vi "labviewArduino_2.vi"() -> ()   [LabVIEW 2017]
uses:
  <vilib>/MakerHub/LINX/Public/Peripherals/Digital/Digital Write N Chans.vi
  <vilib>/MakerHub/LINX/Private/Local IO/LinxDigitalWrite.vi
  <vilib>/MakerHub/LINX/Public/Utilities/Check Channel.vi
  <vilib>/MakerHub/LINX/Public/Utilities/Open Serial.vi
  <vilib>/MakerHub/LINX/Private/Utilties/Generate Error.vi
  Keithley 24XX/Public/Data/Read (Multiple Points).vi
  <vilib>/Utility/file.llb/Write To Spreadsheet File (DBL).vi
  <vilib>/MakerHub/LINX/LMH-LINX.lvlib
  Keithley 24XX/Keithley 24XX.lvlib
panel:
  in  "Tab Control":enum32{"Settings", "General"}(tab)
  in  "Keithley 2400 Cluster":T1={"Compliance  Level (1)"=1.0, "Number of Points (80)"=80, "Minimum Voltage (-0,1)"=-0.1, "Maximum Voltage (0,7)"=0.7, "Timeout (10000 ms)"=100000, "Keithley 2400 GPIB"="", "Source Mode  (0: Voltage)"=0} {"Source Mode  (0: Voltage)" items=["Voltage", "Current"]; "Timeout (10000 ms)" format="%#.6g"}
  in  "HV-Source Cluster":T2={"Control Mode (T = CV, F = CC)"=TRUE, "CH1 ON/OFF (T = ON)"=FALSE, "CH2 ON/OFF (T = ON)"=FALSE, "CH1 VOLTAGE SET (-2000...0 V)"=0, "CH2 VOLTAGE SET (0...+2000 V)"=0, "CH1 CURRENT SET (0...5 mA)"=5.0, "CH2 CURRENT SET (0...5 mA)"=5.0, "COM Port HV Source"=""} {"CH2 CURRENT SET (0...5 mA)" min=0.0 max=5.0 step=0.1 format="%_4f"; "CH1 CURRENT SET (0...5 mA)" min=0.0 max=5.0 step=0.1 format="%_4f"; "CH2 VOLTAGE SET (0...+2000 V)" min=0 max=2000 step=100; "CH1 VOLTAGE SET (-2000...0 V)" min=-2000 max=0 step=100}
  in  "Switch matrix Cluster":T3={"Switch Matrix Port"="", "High voltage Source polarity"=enum."Not inverted", "Total time High Voltage Source is active (min)"=10.0, " Time between measurements(min)"=5.0, "Amount of modules connected"=enum."1", "path to folder for measuring data"=path "C:/Users/Jorne/Documents/Steering Switch matrix/LabVIEW-Masterproef/data", "Stressed time"=0.0}
  in  "Resume Button":bool
  in  "Stop Button 2":bool
  in  "Start Button":bool
  out "Dark IV curve last measurement":cluster{"Voltage":sgl[], "Current":sgl[]}(graph)
  out "Panel measuring":dbl
  out "Total time(s)":dbl
  out "Stressed time (min)":dbl
  in  "Pauze Button":bool
  in  "HV Source emergency STOP)":bool
  out "Last Rsh (Ohm)":dbl
  out "output Rsh":dbl[][](array[numeric])
  out "Rsh curve over time":cluster{"array":dbl[], "array":dbl[]}(graph)
  # "CURE toevoegen: na de stresstijd een curetijd ingeven\nde naam van de opslagbestanden moet dan ook aangepast?\nbutton voor wel of niet curen"
  # "Pauze knop, als erop wordt gedrukt, stopt het stressen en wanneer er terug op start wordt gedrukt, dan start het programma terug van waar het was gestopt"
  # "interface pimpen, met mooiere indeling en greyed out buttons"
  # "Keithley 2400 Setup"
  # "HV Source Setup"
  # "Switch Matrix Setup"
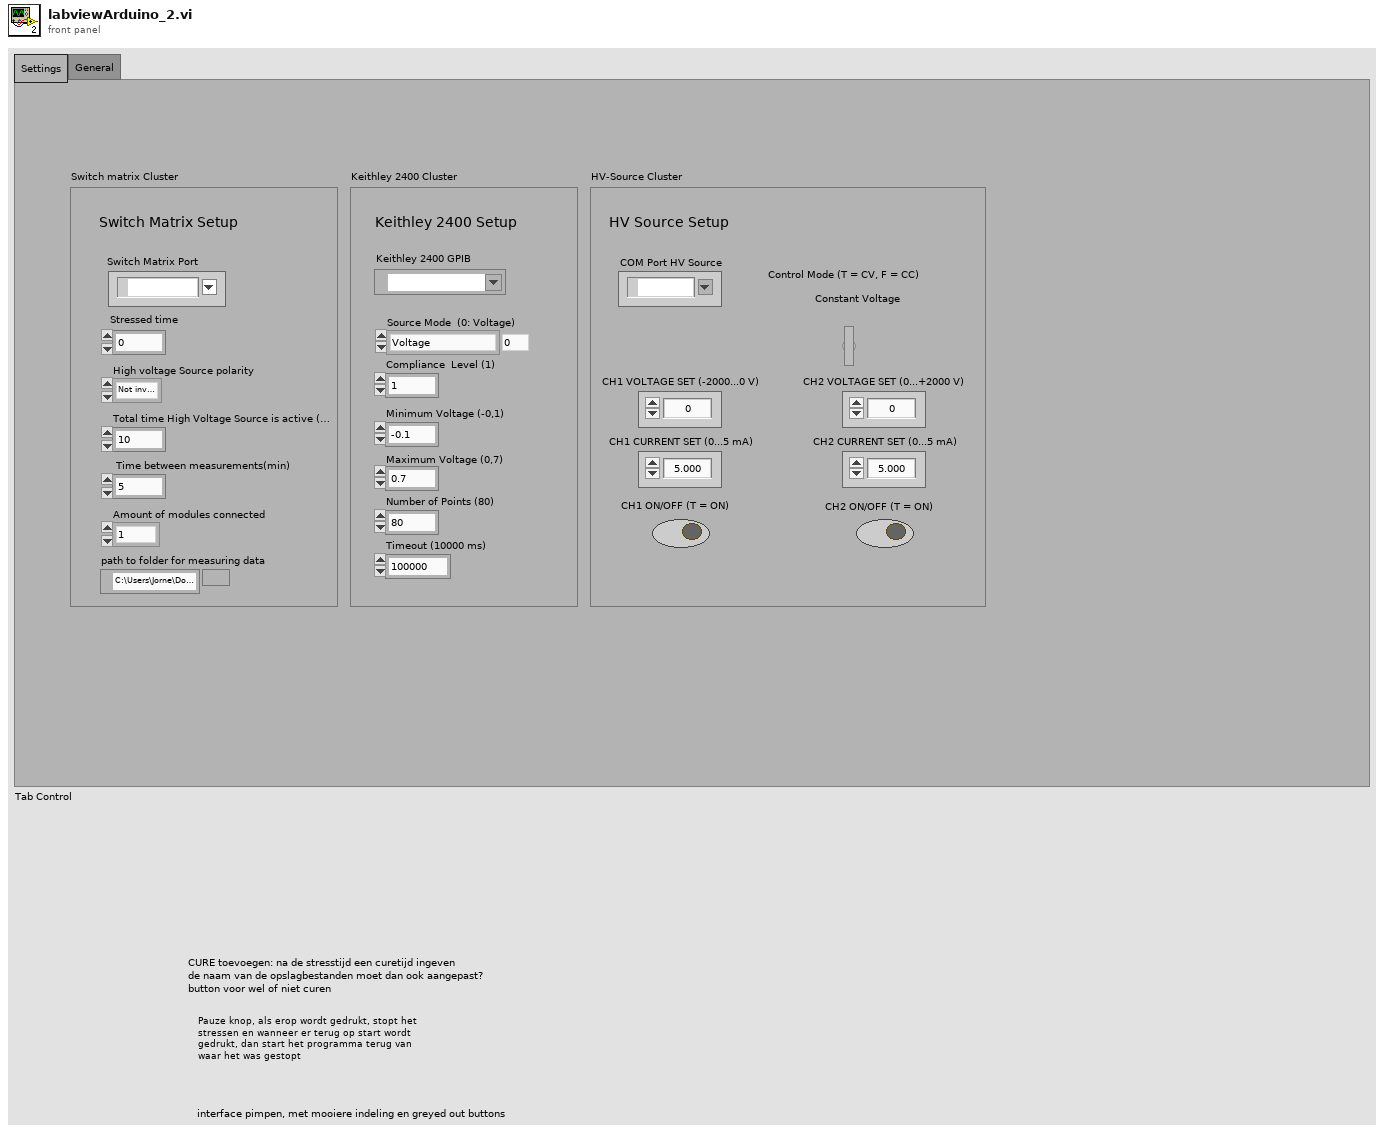
[diagram p1: front panel]
types:
  T1 = cluster{"Compliance  Level (1)":dbl, "Number of Points (80)":u32, "Minimum Voltage (-0,1)":dbl, "Maximum Voltage (0,7)":dbl, "Timeout (10000 ms)":i32, "Keithley 2400 GPIB":refnum<visa-resource-name>, "Source Mode  (0: Voltage)":u16}
  T2 = cluster{"Control Mode (T = CV, F = CC)":bool, "CH1 ON/OFF (T = ON)":bool, "CH2 ON/OFF (T = ON)":bool, "CH1 VOLTAGE SET (-2000...0 V)":i16, "CH2 VOLTAGE SET (0...+2000 V)":i16, "CH1 CURRENT SET (0...5 mA)":dbl, "CH2 CURRENT SET (0...5 mA)":dbl, "COM Port HV Source":refnum<visa-resource-name>}
  T3 = cluster{"Switch Matrix Port":refnum<visa-resource-name>, "High voltage Source polarity":enum16{"Not inverted", "Inverted"}, "Total time High Voltage Source is active (min)":dbl, " Time between measurements(min)":dbl, "Amount of modules connected":enum16{"1", "2", "3", "4", "5", "6"}, "path to folder for measuring data":path, "Stressed time":dbl}
  T4 = enum8{"Enabled", "Disabled", "Disabled and Grayed Out"}
  T5 = enum16{"Rest", "HV Source On", "Measure", "Relay 1", "Relay 2", "Relay 3", "Relay 4", "Relay 5", "Relay 6"}
  T6 = enum16{"Rest", "HV Source On", "Relay 1", "Relay 2", "Relay 3", "Relay 4", "Relay 5", "Relay 6"}
  T7 = typedef "LMH-LINX.lvlib/LINX Ref.ctl" = cluster{"IO":T8, "Interface":T9, "LINX Device Config":T10}
  T8 = typedef "LMH-LINX.lvlib/Platform.ctl" = enum16{"Remote", "Local"}
  T9 = typedef "LMH-LINX.lvlib/Interface.ctl" = enum16{"Serial", "TCP"}
  T10 = typedef "LMH-LINX.lvlib/Device.lvlib/LINX Device Config.ctl" = cluster{"Interface":T9, "COM Port":refnum<visa-resource-name>, "TCP Configuration":T11, "Device Family":u8, "Device ID":u8, "Device Name":string, "TCP Ref":refnum<k5>, "Channels":T12}
  T11 = typedef "LMH-LINX.lvlib/Device.lvlib/TCP Config.ctl" = cluster{"IP Address":string, "Port":u16}
  T12 = typedef "LMH-LINX.lvlib/Channels.ctl" = cluster{"DI":u8[], "DO":u8[], "AI":u8[], "AO":u8[], "PWM":u8[], "QE":u8[], "UART":u8[], "I2C 2":u8[], "SPI":u8[], "CAN":u8[], "Servo":u8[], "AI Ref (V)":dbl, "AI Resolution (Bits)":u8, "AO Ref (V)":dbl, "AO Resolution (Bits)":u8}
  T13 = cluster{"Baud Rate":u32, "Parity":u16, "Data Bits":u16, "Stop Bits":u16, "Flow Control":u16}
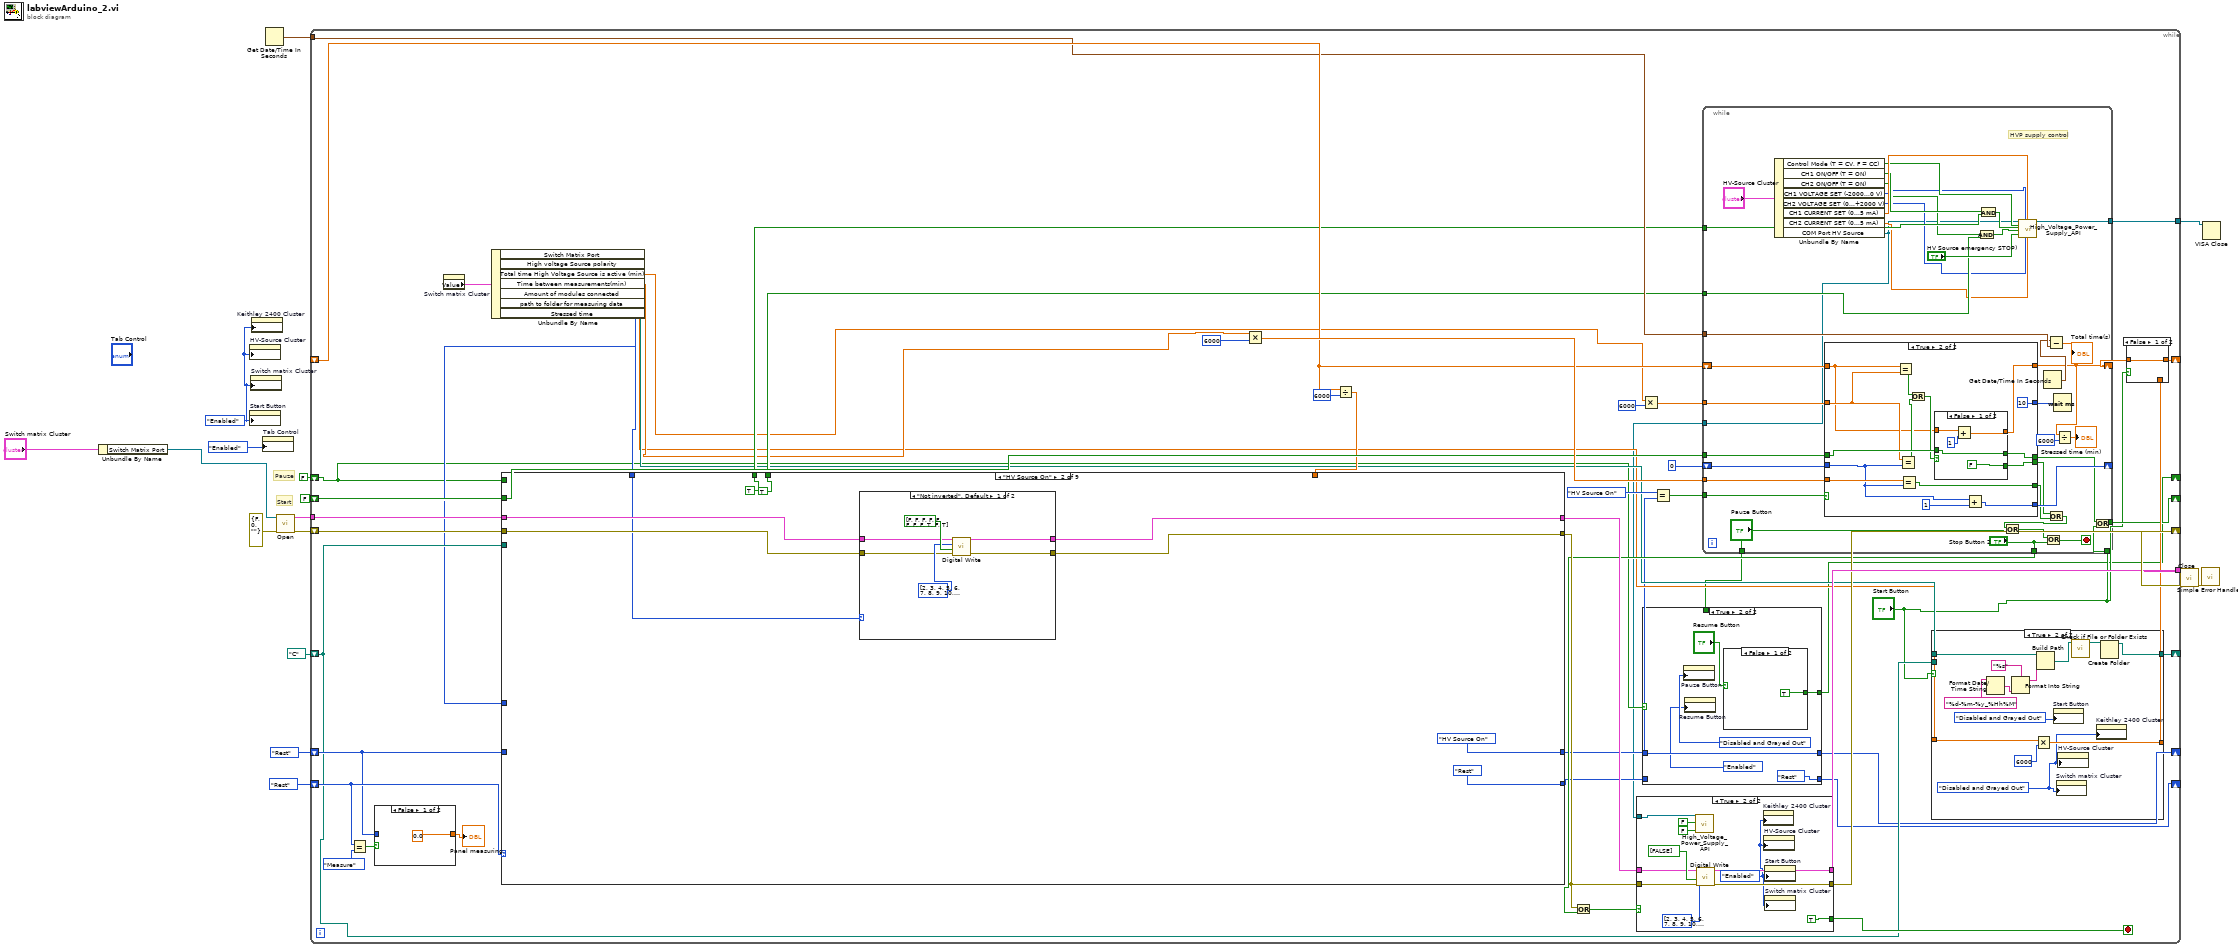
[diagram p0: block diagram]
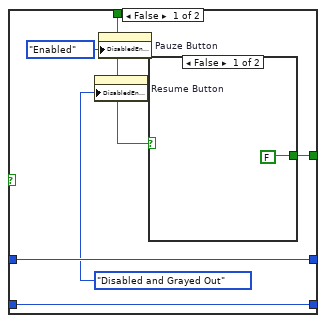
[diagram p2: hidden frame]
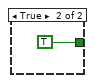
[diagram p3: hidden frame]
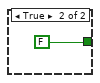
[diagram p4: hidden frame]
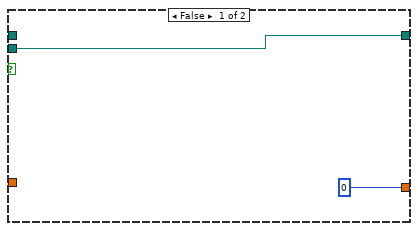
[diagram p6: hidden frame]
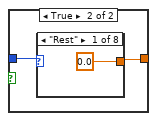
[diagram p7: hidden frame]
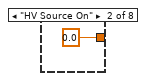
[diagram p8: hidden frame]
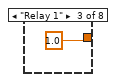
[diagram p9: hidden frame]
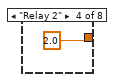
[diagram p10: hidden frame]
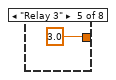
[diagram p11: hidden frame]
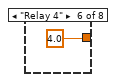
[diagram p12: hidden frame]
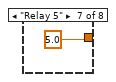
[diagram p13: hidden frame]
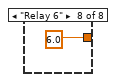
[diagram p14: hidden frame]
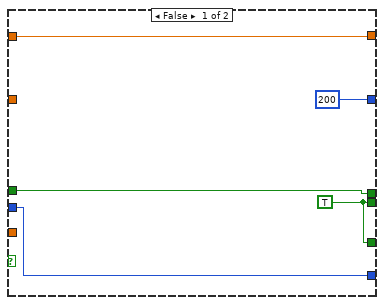
[diagram p15: hidden frame]
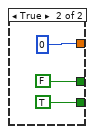
[diagram p16: hidden frame]
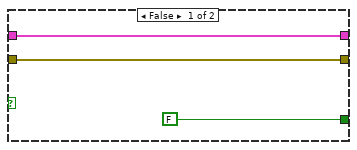
[diagram p17: hidden frame]
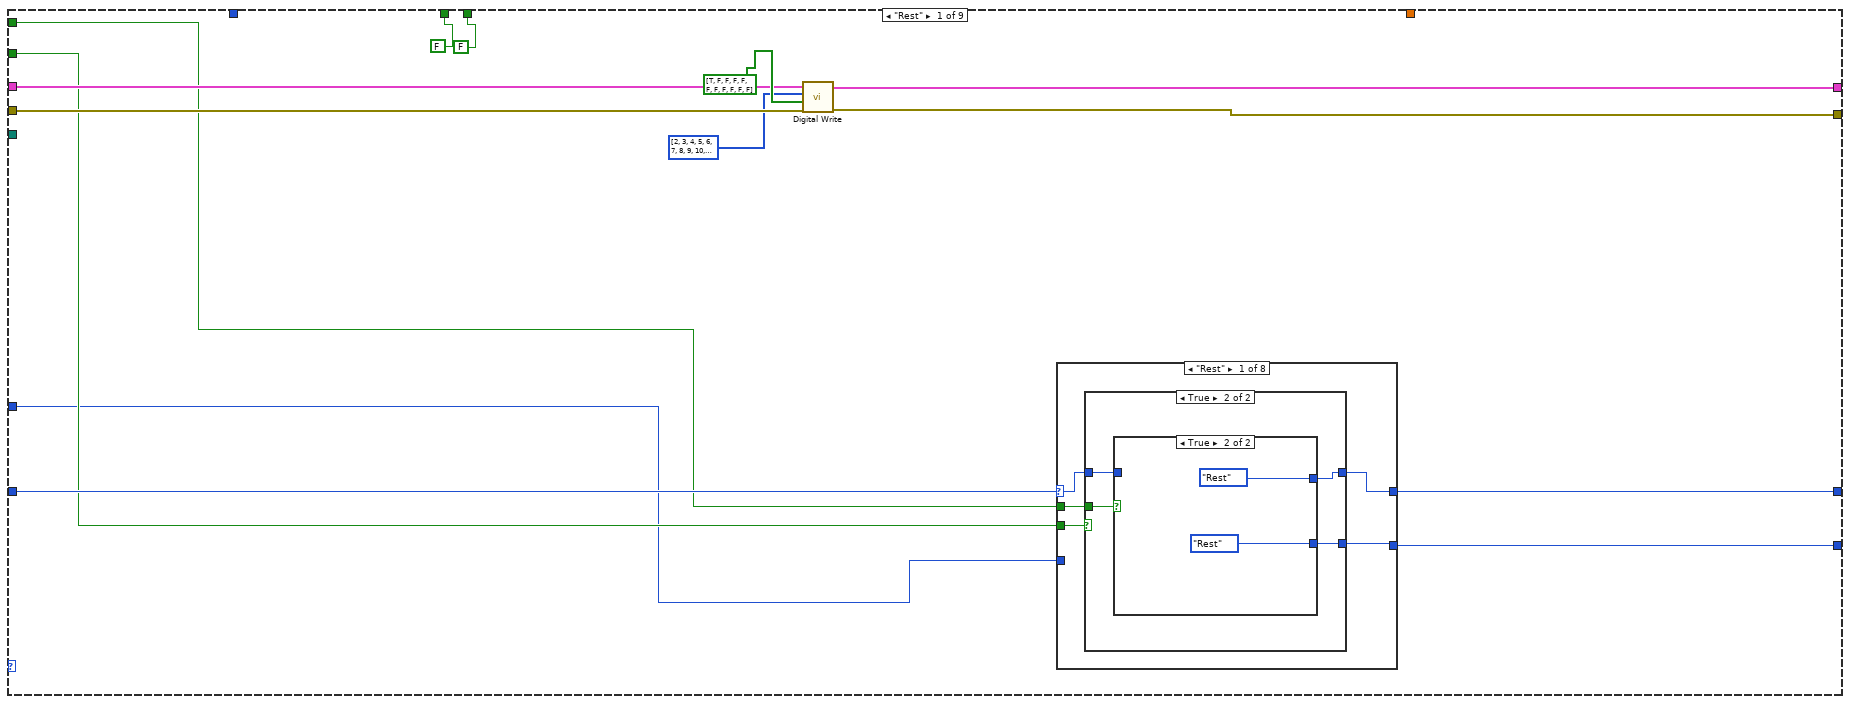
[diagram p18: hidden frame]
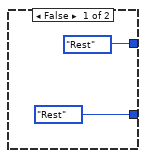
[diagram p19: hidden frame]
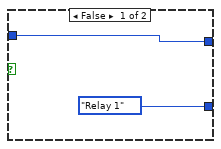
[diagram p20: hidden frame]
diagram:
  w1 = T4."Enabled" ("Disabled")
  # "Start"
  # "Pauze"
  n1 = Unbundle By Name("Switch matrix Cluster") -> ("Switch Matrix Port"=w4:refnum<visa-resource-name>)
  n2 = property on="HV-Source Cluster" class="Clust (strict)"("DisabledEnum"=w1) -> ()  [unwired: 2 in, 2 out]
  n3 = property on="Start Button" class="Bool"("DisabledEnum"=w1) -> ()  [unwired: 2 in, 2 out]
  n4 = property on="Switch matrix Cluster" class="Clust (strict)"("DisabledEnum"=w1) -> ()  [unwired: 2 in, 2 out]
  n5 = property on="Keithley 2400 Cluster" class="Clust (strict)"("DisabledEnum"=w1) -> ()  [unwired: 2 in, 2 out]
  n6 = property on="Tab Control" class="TabCtl (strict)"("DisabledEnum"=T4."Enabled" ("Disabled")) -> ()  [unwired: 2 in, 2 out]
  n7 = Get Date/Time In Seconds() -> (seconds since 1Jan1904=w8:timestamp)
  n8 = call-poly <vilib>:"Open.vi"("Error In"=errorcluster {"status"=FALSE, "code"=0, "source"=""}, "Serial Port"=w4) -> ("Error Out"=w16:errorcluster, "LINX Resource"=w17:T7)  [unwired: 7 in, 1 out]
  n9 = while {
    tunnel: w17 -> [w68]
    tunnel: [w63] -> w15
    shift-right: [w62] -> w14
    shift-left: w16 -> [w67]
    shift-right: [w24] -> _
    shift-left: T5."Rest" ("Enum 2") -> [w49]
    shift-right: [w27] -> _
    shift-left: T6."Rest" ("Enum 2") -> [w46]
    shift-right: [w32] -> _
    shift-left: _ -> [w52]
    shift-right: [w23] -> _
    shift-left: FALSE -> [w53]
    tunnel: w8 -> [w44]
    shift-right: [w42] -> _
    shift-left: path "C:/" ("created path") -> [w41]
    tunnel: [w29] -> w3
    shift-right: [w19] -> _
    shift-left: FALSE -> [w21]
    stop <- w45 stop-if-true
    n10 = Equal?(x=w49, y=T5."Measure") -> (x = y?=w50:bool)
    n11 = case shown="False" w50 {
      tunnel: [0.0 ("Panel measuring") w103] -> w47
      tunnel: w46 -> [_ w104]
      frame False {
      }
      frame True {
        n12 = case shown="\"Rest\"" w104 {
          tunnel: [0.0 ("Panel measuring") 0.0 ("Panel measuring") 1.0 ("Panel measuring") 2.0 ("Panel measuring") 3.0 ("Panel measuring") 4.0 ("Panel measuring") 5.0 ("Panel measuring") 6.0 ("Panel measuring")] -> w103
          frame "Rest" {
          }
          frame "HV Source On" {
          }
          frame "Relay 1" {
          }
          frame "Relay 2" {
          }
          frame "Relay 3" {
          }
          frame "Relay 4" {
          }
          frame "Relay 5" {
          }
          frame "Relay 6" {
          }
        }
      }
    }
    "Panel measuring" <- w47
    n13 = property on="Switch matrix Cluster" class="Clust (strict)"() -> ("Value"=w38:T3)  [unwired: 2 in, 2 out]
    n14 = Unbundle By Name(w38) -> ("High voltage Source polarity"=w37:enum16{"Not inverted", "Inverted"}, "Total time High Voltage Source is active (min)"=w36:dbl, "Time between measurements(min)"=w35:dbl, "Amount of modules connected"=w33:enum16{"1", "2", "3", "4", "5", "6"}, "path to folder for measuring data"=w34:path, "Stressed time"=w28:dbl)  [unwired: 1 out]
    n15 = Multiply(x=w35, y=u32 6000) -> (x*y=w54:dbl)
    n16 = Divide(x=w52, y=u32 6000) -> (x/y=w43:dbl)
    n17 = case shown="\"HV Source On\"" w49 {
      tunnel: [w207 T5."Rest" ("Enum 2") T5."Rest" ("Enum 2") T5."Measure" ("Enum 2") T5."Measure" ("Enum 2") T5."Measure" ("Enum 2") T5."Measure" ("Enum 2") T5."Measure" ("Enum 2") T5."Measure" ("Enum 2")] -> w25
      tunnel: w68 -> [w205 w341 w413 w440 w448 w460 w470 w480 w490]
      tunnel: w67 -> [w204 w340 w412 w439 w447 w459 w469 w479 w489]
      tunnel: [w203 w339 w412 w438 w449 w458 w467 w478 w488] -> w64
      tunnel: [w202 w337 w413 w437 w450 w457 w468 w477 w487] -> w65
      tunnel: [w200 T6."HV Source On" ("Enum 2") w374 T6."Relay 1" ("Enum 2") T6."Relay 2" ("Enum 2") T6."Relay 3" ("Enum 2") T6."Relay 4" ("Enum 2") T6."Relay 5" ("Enum 2") T6."Relay 6" ("Enum 2")] -> w26
      tunnel: w46 -> [w201 _ w374 _ _ _ _ _ _]
      tunnel: w53 -> [w199 _ _ _ _ _ _ _ _]
      tunnel: w43 -> [_ _ w355 _ _ _ _ _ _]
      tunnel: w41 -> [_ _ w367 _ _ _ _ _ _]
      tunnel: [FALSE TRUE FALSE FALSE FALSE FALSE FALSE FALSE FALSE] -> w39
      tunnel: [FALSE TRUE FALSE FALSE FALSE FALSE FALSE FALSE FALSE] -> w40
      tunnel: w37 -> [_ w333 _ _ _ _ _ _ _]
      tunnel: w33 -> [w195 _ _ _ _ _ _ _ _]
      tunnel: w21 -> [w194 _ _ _ _ _ _ _ _]
      frame "Rest" {
        n18 = call-poly <vilib>:"Digital Write.vi"("Error In"=w204, "Values"=bool[] [TRUE, FALSE, FALSE, FALSE, FALSE, FALSE, FALSE, FALSE, FALSE, FALSE, FALSE], "DO Channels"=u8[] [2, 3, 4, 5, 6, 7, 8, 9, 10, 11, 12, 13], "LINX Resource"=w205) -> ("Error Out"=w203:errorcluster, "LINX Resource"=w202:T7)  [unwired: 6 in]
        n19 = case shown="\"Rest\"" w201 {
          selector: w201 -> [w211 _ w227 w246 w263 w277 w295 w315]
          tunnel: [w209 T5."Rest" ("Enum 2") w226 w243 w260 w279 w297 w316] -> w207
          tunnel: [w212 T6."Rest" ("Enum 2") w225 w244 w261 w280 w296 w314] -> w200
          tunnel: w199 -> [w210 _ w228 w245 w262 w278 w294 w313]
          tunnel: w195 -> [_ _ w229 w242 w259 w276 w293 w312]
          tunnel: w194 -> [w208 _ _ _ _ _ _ _]
          frame "Rest" {
            n20 = case shown="True" w210 {
              tunnel: [T6."Rest" ("Enum 2") w217] -> w212
              tunnel: w211 -> [_ w216]
              tunnel: [T5."Rest" ("Enum 2") w218] -> w209
              tunnel: w208 -> [_ w215]
              frame False {
              }
              frame True {
                n21 = case shown="True" w215 {
                  tunnel: [T5."Relay 1" ("Enum 2") T5."Rest" ("Enum 2")] -> w218
                  tunnel: [w220 T6."Rest" ("Enum 2")] -> w217
                  tunnel: w216 -> [w220 _]
                  frame False {
                  }
                  frame True {
                  }
                }
              }
            }
          }
          frame "HV Source On" {
          }
          frame "Relay 1" {
            n22 = Equal?(x=w229, y=enum16{"1", "2", "3", "4", "5", "6"}."1") -> (x = y?=w230:bool)
            n23 = case shown="False" w230 {
              tunnel: [T5."Relay 2" ("Enum 2") w237] -> w226
              tunnel: w227 -> [w233 w236]
              tunnel: [w233 w235] -> w225
              tunnel: w228 -> [_ w234]
              frame False {
              }
              frame True {
                n24 = case shown="False" w234 {
                  tunnel: [T5."Rest" ("Enum 2") T5."HV Source On" ("Enum 2")] -> w237
                  tunnel: [T6."Rest" ("Enum 2") w241] -> w235
                  tunnel: w236 -> [_ w241]
                  frame False {
                  }
                  frame True {
                  }
                }
              }
            }
          }
          frame "Relay 2" {
            n25 = Equal?(x=w242, y=enum16{"1", "2", "3", "4", "5", "6"}."2") -> (x = y?=w247:bool)
            n26 = case shown="False" w247 {
              tunnel: [T5."Relay 3" ("Enum 2") w254] -> w243
              tunnel: w246 -> [w250 w253]
              tunnel: [w250 w252] -> w244
              tunnel: w245 -> [_ w251]
              frame False {
              }
              frame True {
                n27 = case shown="False" w251 {
                  tunnel: [T5."Rest" ("Enum 2") T5."HV Source On" ("Enum 2")] -> w254
                  tunnel: [T6."Rest" ("Enum 2") w258] -> w252
                  tunnel: w253 -> [_ w258]
                  frame False {
                  }
                  frame True {
                  }
                }
              }
            }
          }
          frame "Relay 3" {
            n28 = Equal?(x=w259, y=enum16{"1", "2", "3", "4", "5", "6"}."3") -> (x = y?=w264:bool)
            n29 = case shown="False" w264 {
              tunnel: [T5."Relay 4" ("Enum 2") w271] -> w260
              tunnel: w263 -> [w267 w270]
              tunnel: [w267 w269] -> w261
              tunnel: w262 -> [_ w268]
              frame False {
              }
              frame True {
                n30 = case shown="True" w268 {
                  tunnel: [T5."Rest" ("Enum 2") T5."HV Source On" ("Enum 2")] -> w271
                  tunnel: [T6."Rest" ("Enum 2") w275] -> w269
                  tunnel: w270 -> [_ w275]
                  frame False {
                  }
                  frame True {
                  }
                }
              }
            }
          }
          frame "Relay 4" {
            n31 = Equal?(x=w276, y=enum16{"1", "2", "3", "4", "5", "6"}."4") -> (x = y?=w281:bool)
            n32 = case shown="False" w281 {
              tunnel: [T5."Relay 5" ("Enum 2") w288] -> w279
              tunnel: w277 -> [w284 w287]
              tunnel: [w284 w286] -> w280
              tunnel: w278 -> [_ w285]
              frame False {
              }
              frame True {
                n33 = case shown="False" w285 {
                  tunnel: [T5."Rest" ("Enum 2") T5."HV Source On" ("Enum 2")] -> w288
                  tunnel: [T6."Rest" ("Enum 2") w292] -> w286
                  tunnel: w287 -> [_ w292]
                  frame False {
                  }
                  frame True {
                  }
                }
              }
            }
          }
          frame "Relay 5" {
            n34 = Equal?(x=w293, y=enum16{"1", "2", "3", "4", "5", "6"}."5") -> (x = y?=w298:bool)
            n35 = case shown="False" w298 {
              tunnel: [T5."Relay 6" ("Enum 2") w305] -> w297
              tunnel: w295 -> [w301 w304]
              tunnel: [w301 w303] -> w296
              tunnel: w294 -> [_ w302]
              frame False {
              }
              frame True {
                n36 = case shown="False" w302 {
                  tunnel: [T5."Rest" ("Enum 2") T5."HV Source On" ("Enum 2")] -> w305
                  tunnel: [T6."Rest" ("Enum 2") w309] -> w303
                  tunnel: w304 -> [_ w309]
                  frame False {
                  }
                  frame True {
                  }
                }
              }
            }
          }
          frame "Relay 6" {
            n37 = Equal?(x=w312, y=enum16{"1", "2", "3", "4", "5", "6"}."6") -> (x = y?=w310:bool)
            n38 = case shown="False" w310 {
              tunnel: [w318 w328] -> w316
              tunnel: w315 -> [w320 w327]
              tunnel: [w317 w326] -> w314
              tunnel: w313 -> [w319 w325]
              frame False {
                n39 = case shown="False" w319 {
                  tunnel: [T5."Rest" ("Enum 2") T5."HV Source On" ("Enum 2")] -> w318
                  tunnel: [T6."Rest" ("Enum 2") w324] -> w317
                  tunnel: w320 -> [_ w324]
                  frame False {
                  }
                  frame True {
                  }
                }
              }
              frame True {
                n40 = case shown="False" w325 {
                  tunnel: [T5."Rest" ("Enum 2") T5."HV Source On" ("Enum 2")] -> w328
                  tunnel: [T6."Rest" ("Enum 2") w332] -> w326
                  tunnel: w327 -> [_ w332]
                  frame False {
                  }
                  frame True {
                  }
                }
              }
            }
          }
        }
      }
      frame "HV Source On" {
        n41 = case shown="\"Not inverted\", Default" w333 {
          tunnel: w341 -> [w344 w351]
          tunnel: w340 -> [w345 w350]
          tunnel: [w343 w349] -> w337
          tunnel: [w342 w348] -> w339
          frame "Not inverted", Default {
            n42 = call-poly <vilib>:"Digital Write.vi"("Error In"=w345, "Values"=bool[] [FALSE, FALSE, FALSE, FALSE, FALSE, FALSE, FALSE, FALSE, TRUE, FALSE, TRUE], "DO Channels"=u8[] [2, 3, 4, 5, 6, 7, 8, 9, 10, 11, 12, 13], "LINX Resource"=w344) -> ("Error Out"=w342:errorcluster, "LINX Resource"=w343:T7)  [unwired: 6 in]
          }
          frame "Inverted" {
            n43 = call-poly <vilib>:"Digital Write.vi"("Error In"=w350, "Values"=bool[] [FALSE, FALSE, FALSE, FALSE, FALSE, FALSE, FALSE, FALSE, TRUE, TRUE, TRUE, FALSE], "DO Channels"=u8[] [2, 3, 4, 5, 6, 7, 8, 9, 10, 11, 12, 13], "LINX Resource"=w351) -> ("Error Out"=w348:errorcluster, "LINX Resource"=w349:T7)  [unwired: 6 in]
          }
        }
      }
      frame "Measure" {
        w382 = TRUE  # Enable Output
        w379 = TRUE  # Enable Auto Range
        w378 = u16 1 items=["Volts", "Current", "Resistance"]  # Function
        w377 = u16 0 items=["Volts", "Current", "Resistance"]  # Function
        w381 = FALSE  # Enable Output
        w380 = u16 1 items=["Fixed", "Sweep", "List"]  # Output Mode
        # "Read the raw data.  For the sweep to work correctly, the Output Mode must be set to Sweep."
        # "Configure the sweep with the amplitude and source settings."
        # "Configure the measurements and output."
        n44 = Unbundle By Name("Keithley 2400 Cluster") -> ("Compliance  Level (1)"=w362:dbl, "Number of Points (80)"=w357:u32, "Minimum Voltage (-0,1)"=w361:dbl, "Maximum Voltage (0,7)"=w360:dbl, "Timeout (10000 ms)"=w359:i32, "Keithley 2400 GPIB"=w363:refnum<visa-resource-name>, "Source Mode  (0: Voltage)"=w358:u16)
        n45 = call "Initialize.vi"("Serial Configuration"=T13 {"Baud Rate"=9600, "Parity"=0, "Data Bits"=8, "Stop Bits"=10, "Flow Control"=0}, "VISA resource name"=w363) -> ("error out"=w384:errorcluster, "VISA resource name out"=w383:refnum<visa-resource-name>)  [unwired: 8 in]
        n46 = call "Configure Measurement.vi"("error in (no error)"=w384, "Enable Auto Range (T:Enable)"=w379, "Function (0: Volts)"=w377, "VISA resource name"=w383) -> ("error out"=w385:errorcluster, "VISA resource name out"=w386:refnum<visa-resource-name>)  [unwired: 6 in]
        n47 = call "Configure Measurement.vi"("error in (no error)"=w385, "Enable Auto Range (T:Enable)"=w379, "Function (0: Volts)"=w378, "VISA resource name"=w386) -> ("error out"=w371:errorcluster, "VISA resource name out"=w373:refnum<visa-resource-name>)  [unwired: 6 in]
        n48 = call "Enable Remote Sensing.vi"("error in (no error)"=w371, "Enable Remote Sensing (T: Enable)"=TRUE, "VISA resource name"=w373) -> ("error out"=w370:errorcluster, "VISA resource name out"=w372:refnum<visa-resource-name>)  [unwired: 7 in]
        n49 = call "Configure Output.vi"("Source Mode  (0: Voltage)"=w358, "error in (no error)"=w370, "Compliance  Level (0.1)"=w362, "VISA resource name"=w372) -> ("error out"=w387:errorcluster, "VISA resource name out"=w388:refnum<visa-resource-name>)  [unwired: 6 in]
        n50 = call "Configure Output Sweep.vi"("VISA resource name"=w388, "Source Mode  (0: Voltage)"=w358, "Number of Points (5)"=w357, "Minimum Amplitude (1)"=w361, "Maximum Amplitude (2)"=w360, "error in (no error)"=w387) -> ("VISA resource name out"=w397:refnum<visa-resource-name>, "error out"=w398:errorcluster)  [unwired: 8 in]
        n51 = call "Enable Output.vi"("error in (no error)"=w398, "Enable Output (T: Enable)"=w382, "VISA resource name"=w397) -> ("error out"=w395:errorcluster, "VISA resource name out"=w396:refnum<visa-resource-name>)  [unwired: 7 in]
        n52 = call-poly "Read.vi"("VISA resource name"=w396, "Sample Count (1)"=w357, "Timeout (10000 ms)"=w359, "error in (no error)"=w395, "Output Mode (0: Fixed)"=w380) -> ("Voltage"=w376:sgl[], "VISA resource name out"=w394:refnum<visa-resource-name>, "Current"=w375:sgl[], "error out"=w393:errorcluster)  [unwired: 4 in, 3 out]
        n53 = call "Enable Output.vi"("error in (no error)"=w393, "Enable Output (T: Enable)"=w381, "VISA resource name"=w394) -> ("error out"=w392:errorcluster, "VISA resource name out"=w391:refnum<visa-resource-name>)  [unwired: 7 in]
        n54 = call <vilib>:"Close.vi"("error in (no error)"=w392, "VISA resource name"=w391) -> ("error out"=w390:errorcluster)  [unwired: 9 in]
        n55 = call <vilib>:"Simple Error Handler.vi"("error in (no error)"=w390) -> ()  [unwired: 4 in, 5 out]
        n56 = Build Array(w376, w375) -> (w404:sgl[][])
        n57 = Bundle("Voltage"=w376, "Current"=w375) -> (→"Dark IV curve last measurement":cluster{"Voltage":sgl[], "Current":sgl[]})  [unwired: 1 in]
        n58 = case shown="\"Relay 1\"" w374 {
          tunnel: ["fault" ("name or relative path") "fault" ("name or relative path") "Module1" ("name or relative path") "Module2\\" ("name or relative path") "Module3\\" ("name or relative path") "Module4\\" ("name or relative path") "Module5\\" ("name or relative path") "Module6\\" ("name or relative path")] -> w368
          frame "Rest" {
          }
          frame "HV Source On" {
          }
          frame "Relay 1" {
          }
          frame "Relay 2" {
          }
          frame "Relay 3" {
          }
          frame "Relay 4" {
          }
          frame "Relay 5" {
          }
          frame "Relay 6" {
          }
        }
        n59 = Transpose 2D Array(2D array=w404) -> (transposed array=w354:sgl[][])
        n60 = Build Path(base path=w367, name or relative path=w368) -> (appended path=w407:path)
        n61 = call <vilib>:"Check if File or Folder Exists.vi"("path"=w407) -> ("file or folder exists?"=w406:bool, "dup path"=w356:path)  [unwired: 8 in, 1 out]
        n62 = Format Value(format string="%.;%.0f", value (0)=w355) -> (output string=w411:string)  [unwired: 1 in]
        n63 = case shown="True" w406 {
          tunnel: w356 -> [w418 w422]
          tunnel: [w417 w422] -> w405
          tunnel: w355 -> [w416 w424]
          tunnel: w354 -> [w415 w423]
          frame False {
            n64 = Create Folder(path (use dialog)=w418) -> (created path=w417:path)  [unwired: 2 in, 2 out]
            n65 = call "EmptyCSV.vi"("all rows"=w415, "element"=w416, "base path"=w417) -> ()  [unwired: 8 in, 1 out]
          }
          frame True {
            n66 = call "SavingToExistingCSV.vi"("Numeric"=w424, "all rows"=w423, "base path in"=w422) -> ("output array"=→"output Rsh":dbl[][], "XY Graph 4"=→"Rsh curve over time":cluster{"array":dbl[], "array":dbl[]}, "Last Rsh (Ohm)"=→"Last Rsh (Ohm)":dbl)  [unwired: 5 in, 1 out]
          }
        }
        n67 = Concatenate Strings(w411, ".csv" ("string")) -> (w410:string)
        n68 = Build Path(base path=w405, name or relative path=w410) -> (appended path=w401:path)
        n69 = call-poly <vilib>:"Write To Spreadsheet File.vi"("delimiter (\\t)"=";" ("delimiter (\\t)"), "format (%.3f)"="%.6e", "append to file? (new file:F)"=TRUE, "2D data"=w354, "file path (dialog if empty)"=w401) -> ()  [unwired: 3 in, 1 out]
      }
      frame "Relay 1" {
        n70 = call-poly <vilib>:"Digital Write.vi"("Error In"=w439, "Values"=bool[] [FALSE, TRUE, FALSE, FALSE, FALSE, FALSE, FALSE, TRUE, FALSE, FALSE, FALSE], "DO Channels"=u8[] [2, 3, 4, 5, 6, 7, 8, 9, 10, 11, 12, 13], "LINX Resource"=w440) -> ("Error Out"=w438:errorcluster, "LINX Resource"=w437:T7)  [unwired: 6 in]
      }
      frame "Relay 2" {
        n71 = call-poly <vilib>:"Digital Write.vi"("Error In"=w447, "Values"=bool[] [FALSE, FALSE, TRUE, FALSE, FALSE, FALSE, FALSE, TRUE, FALSE, FALSE, FALSE], "DO Channels"=u8[] [2, 3, 4, 5, 6, 7, 8, 9, 10, 11, 12, 13], "LINX Resource"=w448) -> ("Error Out"=w449:errorcluster, "LINX Resource"=w450:T7)  [unwired: 6 in]
      }
      frame "Relay 3" {
        n72 = call-poly <vilib>:"Digital Write.vi"("Error In"=w459, "Values"=bool[] [FALSE, FALSE, FALSE, TRUE, FALSE, FALSE, FALSE, TRUE, FALSE, FALSE, FALSE], "DO Channels"=u8[] [2, 3, 4, 5, 6, 7, 8, 9, 10, 11, 12, 13], "LINX Resource"=w460) -> ("Error Out"=w458:errorcluster, "LINX Resource"=w457:T7)  [unwired: 6 in]
      }
      frame "Relay 4" {
        n73 = call-poly <vilib>:"Digital Write.vi"("Error In"=w469, "Values"=bool[] [FALSE, FALSE, FALSE, FALSE, TRUE, FALSE, FALSE, TRUE, FALSE, FALSE, FALSE], "DO Channels"=u8[] [2, 3, 4, 5, 6, 7, 8, 9, 10, 11, 12, 13], "LINX Resource"=w470) -> ("Error Out"=w467:errorcluster, "LINX Resource"=w468:T7)  [unwired: 6 in]
      }
      frame "Relay 5" {
        n74 = call-poly <vilib>:"Digital Write.vi"("Error In"=w479, "Values"=bool[] [FALSE, FALSE, FALSE, FALSE, FALSE, TRUE, FALSE, TRUE, FALSE, FALSE, FALSE], "DO Channels"=u8[] [2, 3, 4, 5, 6, 7, 8, 9, 10, 11, 12, 13], "LINX Resource"=w480) -> ("Error Out"=w478:errorcluster, "LINX Resource"=w477:T7)  [unwired: 6 in]
      }
      frame "Relay 6" {
        n75 = call-poly <vilib>:"Digital Write.vi"("Error In"=w489, "Values"=bool[] [FALSE, FALSE, FALSE, FALSE, FALSE, FALSE, TRUE, TRUE, FALSE, FALSE, FALSE], "DO Channels"=u8[] [2, 3, 4, 5, 6, 7, 8, 9, 10, 11, 12, 13], "LINX Resource"=w490) -> ("Error Out"=w488:errorcluster, "LINX Resource"=w487:T7)  [unwired: 6 in]
      }
    }
    n76 = Multiply(x=w36, y=u32 6000) -> (x*y=w56:dbl)
    n77 = Equal?(x=T6."HV Source On", y=w26) -> (x = y?=w60:bool)
    n78 = while {
      tunnel: w60 -> [w151]
      tunnel: w56 -> [w150]
      shift-right: [w148] -> _
      shift-left: u32 0 ("Starting time") -> [w147]
      tunnel: ["Stop Button 2"] -> w58
      tunnel: w54 -> [w144]
      tunnel: w53 -> [w141]
      shift-right: [w134] -> w31
      shift-left: w52 -> [w140]
      tunnel: w44 -> [w138]
      tunnel: w40 -> [w129]
      tunnel: w39 -> [w130]
      tunnel: [w128] -> w29
      tunnel: ["Pauze Button"] -> w20
      tunnel: "Start Button" -> [w116]
      tunnel: [w114] -> w23
      tunnel: [w113] -> w18
      stop <- w146 stop-if-true
      # "HVP supply control"
      n79 = Unbundle By Name("HV-Source Cluster") -> ("Control Mode (T = CV, F = CC)"=w123:bool, "CH1 ON/OFF (T = ON)"=w125:bool, "CH2 ON/OFF (T = ON)"=w124:bool, "CH1 VOLTAGE SET (-2000...0 V)"=w122:i16, "CH2 VOLTAGE SET (0...+2000 V)"=w121:i16, "CH1 CURRENT SET (0...5 mA)"=w126:dbl, "CH2 CURRENT SET (0...5 mA)"=w120:dbl, "COM Port HV Source"=w113:refnum<visa-resource-name>)
      n80 = case shown="True" w151 {
        tunnel: [u32 200 ("millisecond multiple") u32 10 ("millisecond multiple")] -> w149
        tunnel: w150 -> [_ w162]
        tunnel: w147 -> [w155 w167]
        tunnel: [w154 w165] -> w143
        tunnel: [w155 w169] -> w148
        tunnel: w144 -> [_ w168]
        tunnel: [w154 w166] -> w142
        tunnel: [w153 w164] -> w115
        tunnel: w141 -> [w153 w163]
        tunnel: w140 -> [w152 w157]
        tunnel: [w152 w158] -> w134
        frame False {
          w154 = TRUE
        }
        frame True {
          n81 = Equal?(x=w157, y=w162) -> (x = y?=w161:bool)
          n82 = Equal?(x=w162, y=w167) -> (x = y?=w159:bool)
          n83 = Equal?(x=w168, y=w167) -> (x = y?=w166:bool)
          n84 = Or(x=w161, y=w159) -> (x .or. y?=w160:bool)
          n85 = case shown="False" w160 {
            tunnel: [FALSE TRUE] -> w165
            tunnel: [w175 FALSE] -> w164
            tunnel: w163 -> [w175 _]
            tunnel: [w174 0] -> w158
            tunnel: w157 -> [w173 _]
            frame False {
              n86 = Add(x=w173, y=u32 1 ("millisecond multiple")) -> (x+y=w174:dbl)
            }
            frame True {
            }
          }
          n87 = Add(x=w167, y=1) -> (x+y=w169:u32)
        }
      }
      n88 = And(x=w124, y=w130) -> (x .and. y?=w132:bool)
      n89 = And(x=w125, y=w129) -> (x .and. y?=w131:bool)
      n90 = call "High_Voltage_Power_Supply_API.vi"("COM Port In"=w113, "Control Mode (T = CV, F = CC)"=w123, "CH1 ON/OFF (T = ON)"=w131, "CH2 ON/OFF (T = ON)"=w132, "STOP (T = stop)"="HV Source emergency STOP)", "CH1 VOLTAGE SET (-2000...0 V)"=w122, "CH2 VOLTAGE SET (0...+2000 V)"=w121, "CH1 CURRENT SET (0...5 mA)"=w126, "CH2 CURRENT SET (0...5 mA)"=w120) -> ("COM Port Out"=w128:refnum<visa-resource-name>)  [unwired: 11 in, 7 out]
      n91 = Get Date/Time In Seconds() -> (seconds since 1Jan1904=w137:timestamp)
      n92 = Subtract(x=w137, y=w138) -> (x-y=→"Total time(s)":dbl)
      n93 = Or(x=w143, y=w142) -> (x .or. y?=w118:bool)
      n94 = Or(x=w118, y="Pauze Button") -> (x .or. y?=w119:bool)
      n95 = Or(x=w119, y="Stop Button 2") -> (x .or. y?=w146:bool)
      n96 = Wait (ms)(milliseconds to wait=w149) -> ()  [unwired: 1 out]
      n97 = Divide(x=w134, y=u32 6000) -> (x/y=→"Stressed time (min)":dbl)
      n98 = Or(x=w115, y=w116) -> (x .or. y?=w114:bool)
    }
    n99 = Or(x=w64, y=w58) -> (x .or. y?=w66:bool)
    n100 = case shown="True" w66 {
      tunnel: w65 -> [w182 w191]
      tunnel: [w182 w190] -> w63
      tunnel: [w181 w189] -> w62
      tunnel: w64 -> [w181 w188]
      tunnel: [FALSE TRUE] -> w45
      tunnel: w18 -> [_ w183]
      frame False {
      }
      frame True {
        w186 = T4."Enabled" ("Disabled")
        n101 = call "High_Voltage_Power_Supply_API.vi"("COM Port In"=w183, "CH1 ON/OFF (T = ON)"=FALSE, "CH2 ON/OFF (T = ON)"=FALSE) -> ()  [unwired: 17 in, 8 out]
        n102 = call-poly <vilib>:"Digital Write.vi"("Error In"=w188, "Values"=bool[] [FALSE], "DO Channels"=u8[] [2, 3, 4, 5, 6, 7, 8, 9, 10, 11, 12, 13], "LINX Resource"=w191) -> ("Error Out"=w189:errorcluster, "LINX Resource"=w190:T7)  [unwired: 6 in]
        n103 = property on="Keithley 2400 Cluster" class="Clust (strict)"("DisabledEnum"=w186) -> ()  [unwired: 2 in, 2 out]
        n104 = property on="HV-Source Cluster" class="Clust (strict)"("DisabledEnum"=w186) -> ()  [unwired: 2 in, 2 out]
        n105 = property on="Start Button" class="Bool"("DisabledEnum"=w186) -> ()  [unwired: 2 in, 2 out]
        n106 = property on="Switch matrix Cluster" class="Clust (strict)"("DisabledEnum"=w186) -> ()  [unwired: 2 in, 2 out]
      }
    }
    n107 = case shown="True" w21 {
      tunnel: [w74 w81] -> w27
      tunnel: w26 -> [w74 w81]
      tunnel: [w73 T5."Rest" ("Enum 2")] -> w24
      tunnel: w25 -> [w73 _]
      tunnel: w20 -> [w72 _]
      tunnel: [w71 w79] -> w19
      frame False {
        n108 = property on="Resume Button" class="Bool"("DisabledEnum"=T4."Disabled and Grayed Out" ("Disabled")) -> ()  [unwired: 2 in, 2 out]
        n109 = property on="Pauze Button" class="Bool"("DisabledEnum"=T4."Enabled" ("Disabled")) -> ()  [unwired: 2 in, 2 out]
        n110 = case shown="False" w72 {
          tunnel: [FALSE TRUE] -> w71
          frame False {
          }
          frame True {
          }
        }
      }
      frame True {
        n111 = property on="Pauze Button" class="Bool"("DisabledEnum"=T4."Disabled and Grayed Out" ("Disabled")) -> ()  [unwired: 2 in, 2 out]
        n112 = property on="Resume Button" class="Bool"("DisabledEnum"=T4."Enabled" ("Disabled")) -> ()  [unwired: 2 in, 2 out]
        n113 = case shown="False" "Resume Button" {
          tunnel: [TRUE FALSE] -> w79
          frame False {
          }
          frame True {
          }
        }
      }
    }
    n114 = case shown="True" "Start Button" {
      tunnel: w34 -> [_ w101]
      tunnel: [w88 w99] -> w42
      tunnel: w41 -> [w88 _]
      tunnel: w28 -> [_ w91]
      tunnel: [u32 0 w90] -> w30
      frame False {
      }
      frame True {
        w89 = T4."Disabled and Grayed Out" ("Disabled")
        n115 = Format Date/Time String(time format string (%c)="%d-%m-%y_%Hh%M") -> (date/time string=w96:string)  [unwired: 2 in]
        n116 = Format Into String(format string="%s", w96) -> (resulting string=w94:string)  [unwired: 2 in, 1 out]
        n117 = Multiply(x=w91, y=u32 6000) -> (x*y=w90:dbl)
        n118 = Build Path(base path=w101, name or relative path=w94) -> (appended path=w98:path)
        n119 = property on="Start Button" class="Bool"("DisabledEnum"=T4."Disabled and Grayed Out" ("Disabled")) -> ()  [unwired: 2 in, 2 out]
        n120 = property on="Switch matrix Cluster" class="Clust (strict)"("DisabledEnum"=w89) -> ()  [unwired: 2 in, 2 out]
        n121 = property on="HV-Source Cluster" class="Clust (strict)"("DisabledEnum"=w89) -> ()  [unwired: 2 in, 2 out]
        n122 = call <vilib>:"Check if File or Folder Exists.vi"("path"=w98) -> ("dup path"=w100:path)  [unwired: 8 in, 2 out]
        n123 = property on="Keithley 2400 Cluster" class="Clust (strict)"("DisabledEnum"=w89) -> ()  [unwired: 2 in, 2 out]
        n124 = Create Folder(path (use dialog)=w100) -> (created path=w99:path)  [unwired: 2 in, 2 out]
      }
    }
    n125 = case shown="False" "Start Button" {
      tunnel: [w85 w86] -> w32
      tunnel: w31 -> [w85 _]
      tunnel: w30 -> [_ w86]
      frame False {
      }
      frame True {
      }
    }
  }
  n126 = call <vilib>:"Close.vi"("Error In"=w14, "LINX Resource"=w15) -> ("Error Out"=w13:errorcluster)  [unwired: 9 in]
  n127 = call <vilib>:"Simple Error Handler.vi"("error in (no error)"=w13) -> ()  [unwired: 4 in, 5 out]
  n128 = VISA Close(VISA resource name=w3) -> ()  [unwired: 1 in, 1 out]
